vi "Kinect Shutdown.vi"(8 "error in (no error)":errorcluster, 11 "Device_handle":i64) -> (0 "error out":errorcluster)   [LabVIEW 2017]
uses:
  libkinect_wrapper.dll
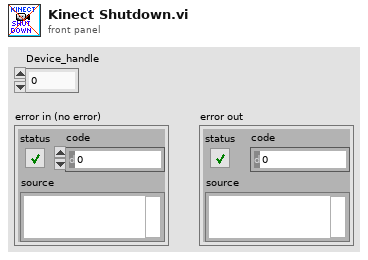
[diagram p1: front panel]
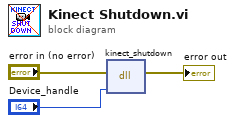
[diagram p0: block diagram]
diagram:
  n1 = dll-call lib="libkinect_wrapper.*" fn="kinect_shutdown"(error in="error in (no error)", "Context_handle"="Device_handle") -> (error out=→"error out":errorcluster)  [unwired: 4 in, 1 out]
